vi "p1.vi"() -> ()   [LabVIEW 2023, in "d24.lvlib"]
uses:
  d24.lvlib
  AOC/AOC.lvlib
panel:
  in  "Example":string
  in  "Example":bool=TRUE
  out "Answer":i64=10
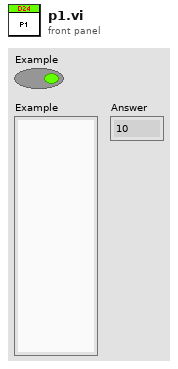
[diagram p1: front panel]
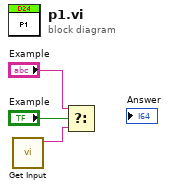
[diagram p0: block diagram]
diagram:
  n1 = call "Get Input.vi"() -> ("Input"=w3:string)  [unwired: 11 in]
  n2 = Select(t="Example", s="Example", f=w3) -> ()  [unwired: 1 out]
